vi "Test MQTT-4.7.1-1.vi"(8 "error in (no error)":errorcluster) -> (0 "error out":errorcluster)   [LabVIEW 2013]
uses:
  <vilib>/addons/_JKI Toolkits/Caraya/classes/Test/Test.lvclass
  <vilib>/addons/_JKI Toolkits/Caraya/classes/Assert/Assert.lvclass
  <vilib>/LabVIEW Open Source Project/MQTT Control Packets/Control Packets/PUBLISH/PUBLISH.lvclass
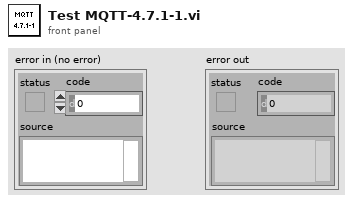
[diagram p1: front panel]
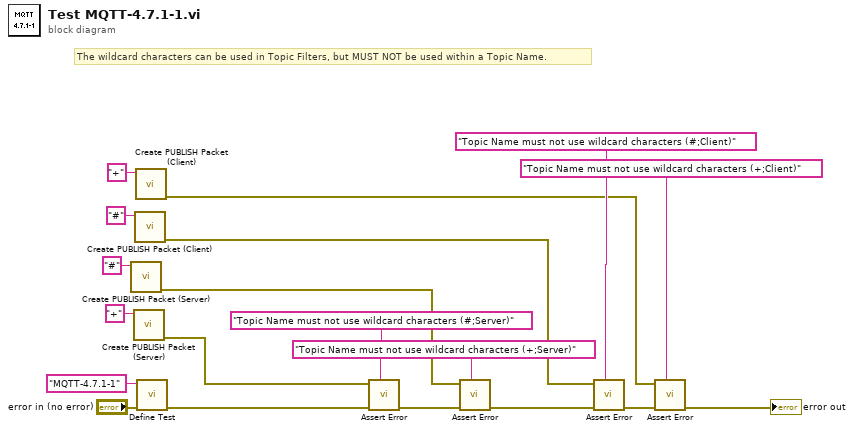
[diagram p0: block diagram]
diagram:
  # "The wildcard characters can be used in Topic Filters, but MUST NOT be used within a Topic Name."
  n1 = call <vilib>:"Create PUBLISH Packet (Server).vi"("Topic Name"="#") -> ("error out"=w3:errorcluster)  [unwired: 7 in, 3 out]
  n2 = call <vilib>:"Create PUBLISH Packet (Server).vi"("Topic Name"="+") -> ("error out"=w15:errorcluster)  [unwired: 7 in, 3 out]
  n3 = call <vilib>:"Create PUBLISH Packet (Client).vi"("Topic Name"="#") -> ("error out"=w13:errorcluster)  [unwired: 7 in, 3 out]
  n4 = call <vilib>:"Create PUBLISH Packet (Client).vi"("Topic Name"="+") -> ("error out"=w7:errorcluster)  [unwired: 7 in, 3 out]
  n5 = call <vilib>:"Define Test.vi"("error in (no error)"="error in (no error)", "Label (VI Title)"="MQTT-4.7.1-1") -> ("error out"=w16:errorcluster)  [unwired: 9 in]
  n6 = call <vilib>:"Assert Error.vi"("Label"="Topic Name must not use wildcard characters (#;Server)", "error in (no error)"=w16, "Error?"=w15) -> ("error out"=w5:errorcluster)  [unwired: 8 in]
  n7 = call <vilib>:"Assert Error.vi"("Label"="Topic Name must not use wildcard characters (+;Server)", "error in (no error)"=w5, "Error?"=w3) -> ("error out"=w4:errorcluster)  [unwired: 8 in]
  n8 = call <vilib>:"Assert Error.vi"("Label"="Topic Name must not use wildcard characters (#;Client)", "error in (no error)"=w4, "Error?"=w13) -> ("error out"=w10:errorcluster)  [unwired: 8 in]
  n9 = call <vilib>:"Assert Error.vi"("Label"="Topic Name must not use wildcard characters (+;Client)", "error in (no error)"=w10, "Error?"=w7) -> ("error out"=→"error out":errorcluster)  [unwired: 8 in]
